vi "Config Type.vi"(11 "State Transition in":refnum<class "State Transition.lvclass">) -> (2 "Config Type":refnum<class "Transition Config.lvclass">)   [LabVIEW 2020, in "VolatusSeq.lvlib" / "State Transition.lvclass"]
uses:
  State Transition.lvclass
  State Transition.lvclass/State Transition.ctl
  VolatusSeqConfig/State Transition Config/State Transition Config.lvclass
  C:/dev/lv20CE/relink/lv-volatus/VolatusSeqConfig/Transition Config/Transition Config.lvclass
  C:/dev/lv20CE/relink/lv-volatus/VolatusSeqConfig/State Transition Config/State Transition Config.lvclass
  VolatusSeqConfig/Transition Config/Transition Config.lvclass
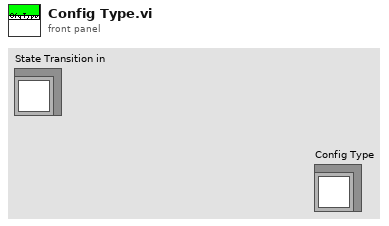
[diagram p1: front panel]
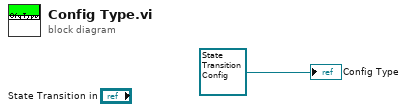
[diagram p0: block diagram]
diagram:
  "Config Type" <- refnum<class "State Transition Config.lvclass"> refnum ("VolatusSeqConfig.lvlib:State Transition Config.lvclass")
